vi "FUG_MagnetPS.ProcPeriodic.vi"(0 "i ref in":refnum<vi>, 3 "ms timeout (10000)":i32=10000, 5 "error in (no error)":errorcluster) -> (14 "i ref out":refnum<vi>, 17 "timed out":bool, 19 "error out":errorcluster)   [LabVIEW 2014, in "FUG_MagnetPS.lvlib"]
doc: "This method serves to periodically do things like reading values from the HW. Methods that should be executed periodically should be called from THIS methode. Add code here."
uses:
  FUG_MagnetPS.lvlib
  CSlibraries-extern/DimLVEvent/LVDimInterface/LVDimInterface.lvlib
  CSPowerSupply/FUG_PowerSupply/FUG_PowerSupply.lvlib
  CSCore/CSApplicationBaseClasses/PSChannelBase/PSChannelBase.lvlib
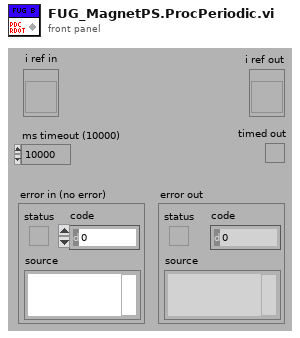
[diagram p1: front panel]
types:
  T1 = typedef "FUG_MagnetPS.lvlib/FUG_MagnetPS.i attribute.ctl" = cluster{"Gaussmeter":string, "SetField":dbl, "MagneticField queue":refnum<queue>, "Field Callback ID":i32, "nomCurrent":dbl, "Proportional":dbl, "Regulation?":bool, "actFieldID":i32, "nomFieldID":i32, "nomAutoCurrentID":i32, "regCurrentID":i32}
  T2 = typedef "PSChannelBase.lvlib/PSChannelBase.i attribute.ctl" = cluster{"defaultChannelIndex":i32, "nofChannels":i32, "defaultChannelIndexID":i32, "nofChannelsID":i32, "actValues":T3, "nomValues":T3, "logicalName":string[], "physicalName":string[], "logicalNameID":i32, "physicalNameID":i32}
  T3 = typedef "PSChannelBase.lvlib/PSChannelBase.parameters.ctl" = cluster{"onOff":bool[], "voltage":dbl[], "current":dbl[], "tripCurrent":dbl[], "rampUpSpeed":dbl[], "rampDownSpeed":dbl[], "status":i32[], "serviceIDs":cluster{"onOfflID":i32, "voltageID":i32, "currentID":i32, "tripCurrentID":i32, "rampUpSpeedID":i32, "rampDownSpeedID":i32, "statusID":i32}}
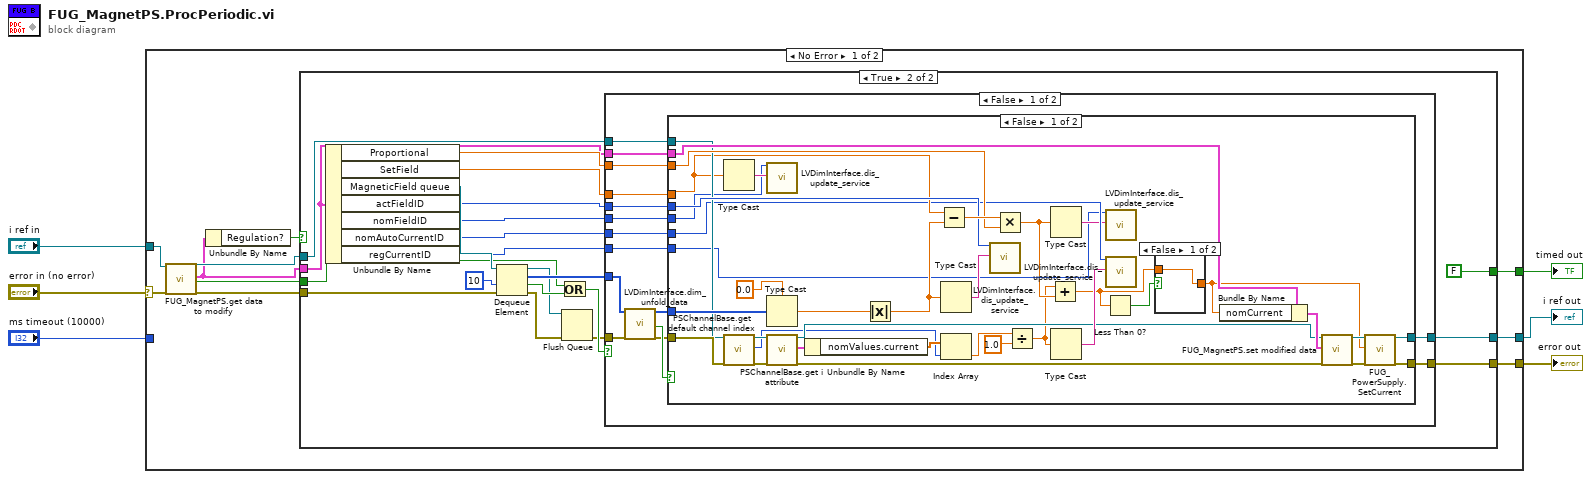
[diagram p0: block diagram]
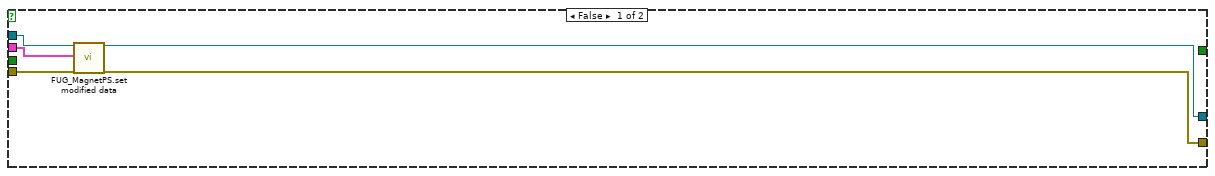
[diagram p2: hidden frame]
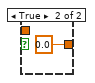
[diagram p3: hidden frame]
diagram:
  n1 = case shown="No Error" "error in (no error)" {
    selector: "error in (no error)" -> [w14 w101]
    tunnel: [w12 w101] -> w5
    tunnel: "i ref in" -> [w15 w102]
    tunnel: [w13 w102] -> w3
    tunnel: [w16 _] -> w2
    tunnel: "ms timeout (10000)" -> [_ _]
    frame No Error {
      n2 = call "FUG_MagnetPS.get data to modify.vi"("i ref in"=w15, "error in (no error)"=w14) -> ("i ref out"=w10:refnum<vi>, "i attribute"=w8:T1, "timed out"=w9:bool, "error out"=w11:errorcluster)  [unwired: 14 in]
      n3 = Unbundle By Name(w8) -> ("Regulation?"=w7:bool)
      n4 = case shown="True" w7 {
        tunnel: [_ FALSE] -> w16
        tunnel: [w17 w41] -> w13
        tunnel: [w18 w40] -> w12
        tunnel: w11 -> [w19 w37]
        tunnel: w10 -> [w20 w33]
        tunnel: w9 -> [_ w30]
        tunnel: w8 -> [w21 w29]
        frame False {
          n5 = call "FUG_MagnetPS.set modified data.vi"("i ref in"=w20, "i attribute"=w21, "error in (no error)"=w19) -> ("i ref out"=w17:refnum<vi>, "error out"=w18:errorcluster)  [unwired: 15 in]
        }
        frame True {
          n6 = Unbundle By Name(w29) -> ("Proportional"=w34:dbl, "SetField"=w35:dbl, "MagneticField queue"=w36:refnum<queue>, "actFieldID"=w28:i32, "nomFieldID"=w24:i32, "nomAutoCurrentID"=w23:i32, "regCurrentID"=w22:i32)
          n7 = Dequeue Element(queue=w36, timeout in ms (-1)=10, error in (no error)=w37) -> (queue out=w25:refnum<queue>, element=w38:i8[], timed out?=w31:bool, error out=w27:errorcluster)
          n8 = Or(x=w30, y=w31) -> (x .or. y?=w32:bool)
          n9 = Flush Queue(queue=w25, error in (no error)=w27) -> (error out=w26:errorcluster)  [unwired: 2 out]
          n10 = case shown="False" w32 {
            tunnel: w38 -> [w57 _]
            tunnel: w26 -> [w56 w100]
            tunnel: w35 -> [w52 _]
            tunnel: w34 -> [w51 _]
            tunnel: w33 -> [w50 w99]
            tunnel: [w49 w99] -> w41
            tunnel: [w48 w100] -> w40
            tunnel: w29 -> [w47 _]
            tunnel: w28 -> [w46 _]
            tunnel: w24 -> [w45 _]
            tunnel: w23 -> [w44 _]
            tunnel: w22 -> [w43 _]
            frame False {
              n11 = call "LVDimInterface.dim_unfold_data.vi"("rawData"=w57, "error in (no error)"=w56) -> ("data"=w55:i8[], "no link"=w54:bool, "error out"=w53:errorcluster)  [unwired: 14 in, 1 out]
              n12 = case shown="False" w54 {
                tunnel: w55 -> [w94 _]
                tunnel: w53 -> [w81 w97]
                tunnel: w52 -> [w74 _]
                tunnel: w51 -> [w89 _]
                tunnel: w50 -> [w80 w98]
                tunnel: [w86 w98] -> w49
                tunnel: [w85 w97] -> w48
                tunnel: w47 -> [w92 _]
                tunnel: w46 -> [w84 _]
                tunnel: w45 -> [w75 _]
                tunnel: w44 -> [w73 _]
                tunnel: w43 -> [w71 _]
                frame False {
                  n13 = Type Cast(x=w74) -> (*(type *) &x=w76:string)  [unwired: 1 in]
                  n14 = call "PSChannelBase.get default channel index.vi"("i ref in"=w80, "error in (no error)"=w81) -> ("i ref out"=w64:refnum<vi>, "defaultChannelIndex"=w60:i32, "error out"=w66:errorcluster)  [unwired: 15 in]
                  n15 = call "LVDimInterface.dis_update_service.vi"("my_serviceID"=w75, "data"=w76) -> ()  [unwired: 15 in, 3 out]
                  n16 = Type Cast(type=0.0, x=w94) -> (*(type *) &x=w82:dbl)
                  n17 = call "PSChannelBase.get i attribute.vi"("i ref in"=w64, "error in (no error)"=w66) -> ("i ref out"=w63:refnum<vi>, "i attribute"=w62:T2, "error out"=w65:errorcluster)  [unwired: 15 in]
                  n18 = Unbundle By Name(w62) -> ("nomValues.current"=w61:dbl[])
                  n19 = Absolute Value(x=w82) -> (abs(x)=w78:dbl)
                  n20 = Subtract(x=w74, y=w78) -> (x-y=w90:dbl)
                  n21 = Type Cast(x=w78) -> (*(type *) &x=w83:string)  [unwired: 1 in]
                  n22 = Index Array(array=w61, index=w60) -> (element=w59:dbl)
                  n23 = call "LVDimInterface.dis_update_service.vi"("my_serviceID"=w84, "data"=w83) -> ()  [unwired: 15 in, 3 out]
                  n24 = Multiply(x=w90, y=w89) -> (x*y=w70:dbl)
                  n25 = Divide(x=w59, y=1.0) -> (x/y=w58:dbl)
                  n26 = Add(x=w58, y=w70) -> (x+y=w68:dbl)
                  n27 = Type Cast(x=w70) -> (*(type *) &x=w72:string)  [unwired: 1 in]
                  n28 = Type Cast(x=w58) -> (*(type *) &x=w77:string)  [unwired: 1 in]
                  n29 = Less Than 0?(x=w68) -> (x < 0?=w69:bool)
                  n30 = call "LVDimInterface.dis_update_service.vi"("my_serviceID"=w71, "data"=w72) -> ()  [unwired: 15 in, 3 out]
                  n31 = call "LVDimInterface.dis_update_service.vi"("my_serviceID"=w73, "data"=w77) -> ()  [unwired: 15 in, 3 out]
                  n32 = case shown="False" w69 {
                    tunnel: w68 -> [w95 _]
                    tunnel: [w95 0.0] -> w67
                    frame False {
                    }
                    frame True {
                    }
                  }
                  n33 = Bundle By Name(cluster=w92, "nomCurrent"=w67) -> (w91:T1)
                  n34 = call "FUG_MagnetPS.set modified data.vi"("i ref in"=w63, "i attribute"=w91, "error in (no error)"=w65) -> ("i ref out"=w87:refnum<vi>, "error out"=w88:errorcluster)  [unwired: 15 in]
                  n35 = call "FUG_PowerSupply.SetCurrent.vi"("i ref in"=w87, "value"=w67, "error in (no error)"=w88) -> ("i ref out"=w86:refnum<vi>, "error out (no error)"=w85:errorcluster)  [unwired: 15 in]
                }
                frame True {
                }
              }
            }
            frame True {
            }
          }
        }
      }
    }
    frame Error {
    }
  }
  "error out" <- w5
  "i ref out" <- w3
  "timed out" <- w2
